vi "Reslut.vi"() -> ()   [LabVIEW 2018]
uses:
  <vilib>/vision/Image Controls.llb/IMAQ Image.ctl
panel:
  out "存储时间":string
  out "Result_Spetrometer":T1
  out "Result_Near/Far":T3
  out "Reslut_Scope":T4
  out "Reslut _PolarMeter":T5
  out "Reslut_Power/Energy":T6
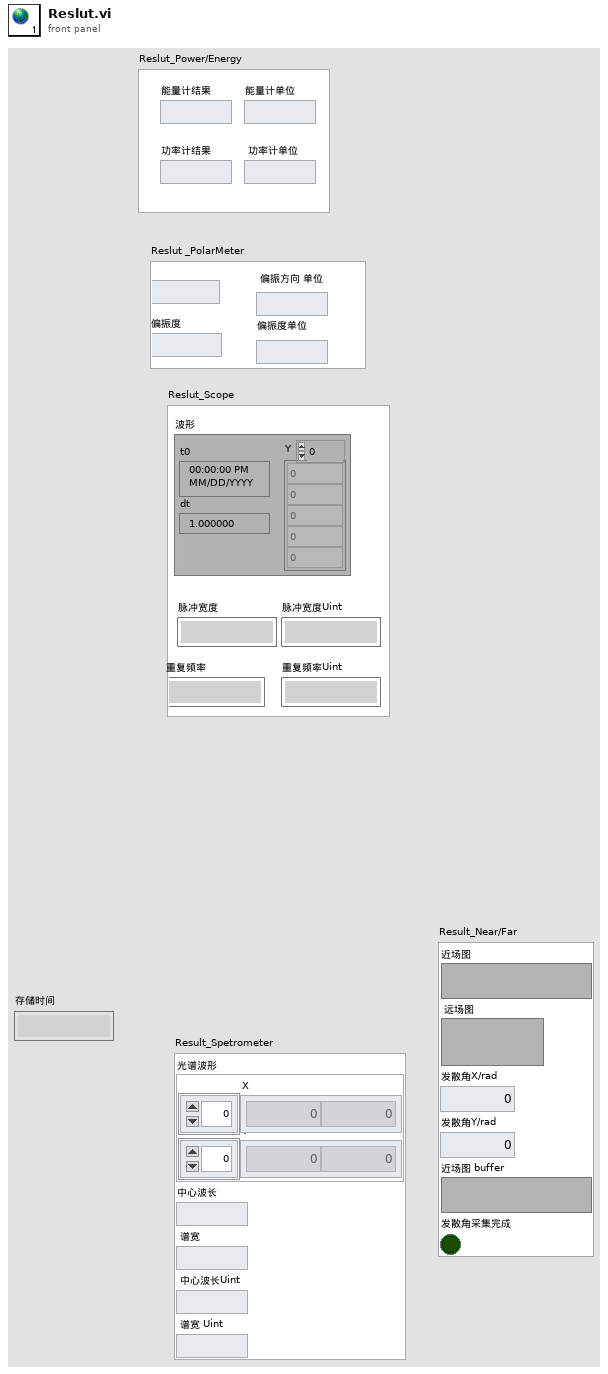
[diagram p1: front panel]
types:
  T1 = cluster{"光谱波形":cluster{"X":dbl[], "Y":dbl[]}, "中心波长":string, " 谱宽":string, " 中心波长Uint":string, " 谱宽 Uint":string}
  T2 = typedef "IMAQ Image.ctl" = refnum<image>
  T3 = cluster{"近场图":T2, " 远场图":T2, "发散角X/rad":dbl, "发散角Y/rad":dbl, "近场图 buffer":T2, "发散角采集完成":bool}
  T4 = cluster{"波形":waveform(dbl), "脉宽":string, "重频":string, "脉冲宽度Uint":string, "重复频率Uint":string}
  T5 = cluster{" 偏振方向":string, "偏振度":string, " 偏振方向 单位 ":string, "偏振度单位":string}
  T6 = cluster{"能量计结果":string, "功率计结果":string, "能量计单位":string, " 功率计单位":string}
diagram:
